vi "Load Maze.vi"(8 "error in (no error)":errorcluster, 11 "Maze File Path (*.maz)":path) -> (0 "error out":errorcluster, 3 "Maze":refnum<class "Maze.lvclass">)   [LabVIEW 2020]
uses:
  Adjacency.ctl
  Maze.lvlib
  Position.ctl
  Maze/Maze.lvclass
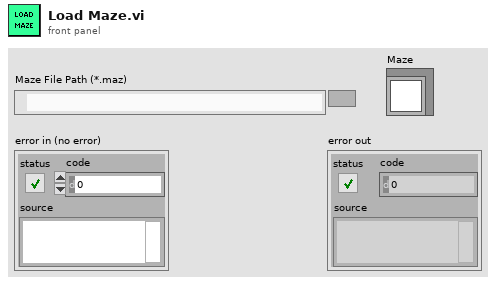
[diagram p1: front panel]
types:
  T1 = typedef "Maze.lvlib/Position.ctl" = cluster{"S":i32, "E":i32}
  T2 = typedef "Maze.lvlib/Adjacency.ctl" = cluster{"E":bool, "N":bool, "W":bool, "S":bool, "Goal":bool, "Start":bool}
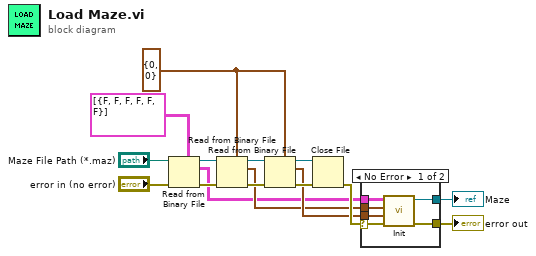
[diagram p0: block diagram]
diagram:
  w9 = T1 {"S"=0, "E"=0} ("Position")
  n1 = Read from Binary File(5:T2[][] [[{"E"=FALSE, "N"=FALSE, "W"=FALSE, "S"=FALSE, "Goal"=FALSE, "Start"=FALSE}]], 8:"error in (no error)", 11:"Maze File Path (*.maz)") -> (0:w12:errorcluster, 2:w2:T2[][], 3:w13:refnum<file>)  [unwired: 3 in, 1 out]
  n2 = Read from Binary File(5:w9, 8:w12, 11:w13) -> (0:w10:errorcluster, 2:w3:T1, 3:w11:refnum<file>)  [unwired: 3 in, 1 out]
  n3 = Read from Binary File(5:w9, 8:w10, 11:w11) -> (0:w7:errorcluster, 2:w4:T1, 3:w8:refnum<file>)  [unwired: 3 in, 1 out]
  n4 = Close File(refnum=w8, error in=w7) -> (error out=w6:errorcluster)  [unwired: 1 out]
  n5 = case shown="No Error" w6 {
    selector: w6 -> [w22 w23]
    tunnel: [w21 _] -> w5
    tunnel: w4 -> [w20 _]
    tunnel: w3 -> [w19 _]
    tunnel: w2 -> [w18 _]
    tunnel: [w17 w23] -> w1
    frame No Error {
      n6 = call "Init.vi"("error in (no error)"=w22, "Goal"=w20, "Start"=w19, "Adjacency"=w18) -> ("error out"=w17:errorcluster, "Maze out"=w21:refnum<class "Maze.lvclass">)  [unwired: 6 in]
    }
    frame Error {
    }
  }
  "Maze" <- w5
  "error out" <- w1
